vi "StringToNumberControlWithBool.vi"(7 "Numeric In":dbl, 9 "String In":string) -> (2 "Number Out":dbl, 4 "NOT = 0":bool)   [LabVIEW 2018]
doc: "Input a String and return a Number.\n\nLeave String blank, and a number returns."
panel:
  out "error out":errorcluster
  in  "error in":errorcluster
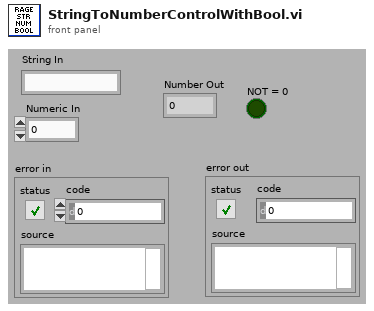
[diagram p1: front panel]
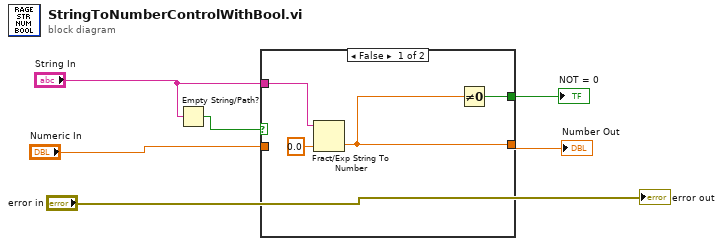
[diagram p0: block diagram]
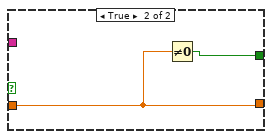
[diagram p2: hidden frame]
diagram:
  n1 = Empty String/Path?(string/path="String In") -> (empty?=w4:bool)
  n2 = case shown="False" w4 {
    tunnel: [w8 w12] -> w6
    tunnel: "Numeric In" -> [_ w12]
    tunnel: "String In" -> [w10 _]
    tunnel: [w7 w11] -> w2
    frame False {
      n3 = Fract/Exp String To Number(string=w10, default (0 dbl)=0.0 ("default (0 DBL)")) -> (number=w8:dbl)  [unwired: 2 in, 1 out]
      n4 = Not Equal To 0?(x=w8) -> (x != 0?=w7:bool)
    }
    frame True {
      n5 = Not Equal To 0?(x=w12) -> (x != 0?=w11:bool)
    }
  }
  "Number Out" <- w6
  "NOT = 0" <- w2
  "error out" <- "error in"
